vi "GE 5565PIORC.PIO.Window.Get Base Address.vi"(8 "error in (no error)":errorcluster, 10 "offset":u32 format="%.0x", 11 "GE 5565PIORC in":refnum<class "GE 5565PIORC.lvclass">) -> (0 "error out":errorcluster, 2 "base address":u32 format="%.0x", 3 "GE 5565PIORC out":refnum<class "GE 5565PIORC.lvclass">)   [LabVIEW 2016, in "GE 5565PIORC.lvclass"]
doc: "Runs the provided <B>offset</B> through a mask, which returns the <B>base address</B> of the PIO window the offset exists within. The PIO Window size is defined by hardware DIP switches on the GE 5565PIORC board, and cannot be changed once powered on."
uses:
  GE 5565PIORC.lvclass
  GE 5565PIORC.lvclass/GE 5565PIORC.ctl
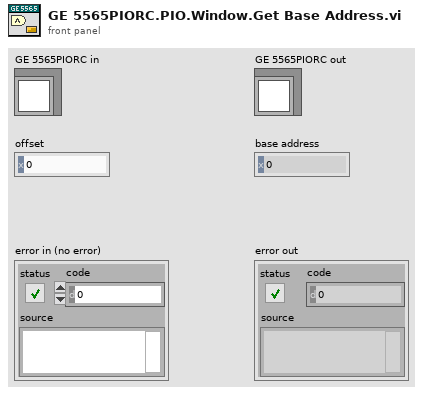
[diagram p1: front panel]
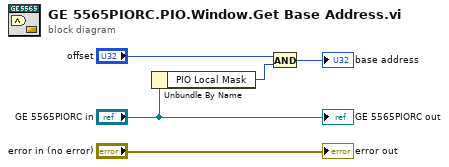
[diagram p0: block diagram]
diagram:
  n1 = Unbundle By Name("GE 5565PIORC in") -> ("PIO Local Mask"=w4:u32)
  n2 = And(x="offset", y=w4) -> (x .and. y?=→"base address":u32)
  "GE 5565PIORC out" <- "GE 5565PIORC in"
  "error out" <- "error in (no error)"
